vi "Queue Driver-Receive.vi"(0 "States[]":string[](array[string]), 5 "Data":variant, 7 "Queue Name":string, 11 "Error In":errorcluster, 13 "Queue Operation":T2) -> (4 "Dequeue Element":T1, 15 "Error Out":errorcluster)   [LabVIEW 2020]
doc: "The VI performs the queue operations. The operations include create, enqueue, dequeue, flush and closes the queue."
uses:
  Controls/Queue Element.ctl
  Controls/Queue Operation.ctl
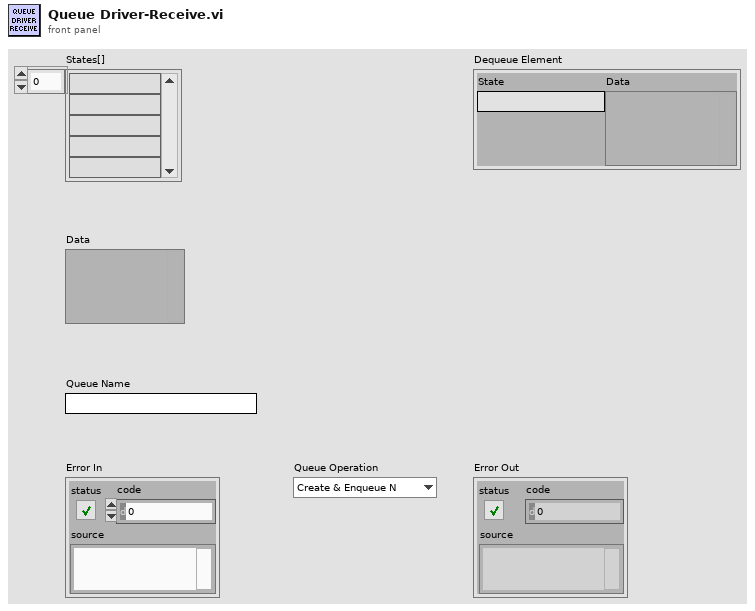
[diagram p1: front panel]
types:
  T1 = typedef "Queue Element.ctl" = cluster{"State":string, "Data":variant}
  T2 = typedef "Queue Operation.ctl" = enum16{"Create & Enqueue N", "Enqueue N", "Dequeue", "Enstack N", "Flush", "Release"}
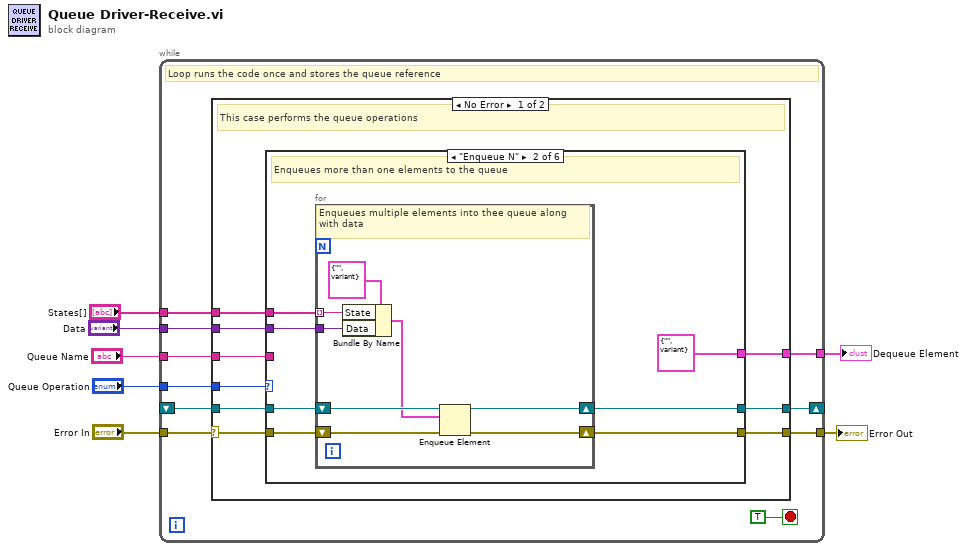
[diagram p0: block diagram]
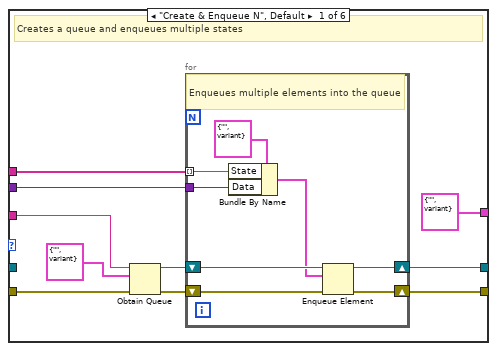
[diagram p2: hidden frame]
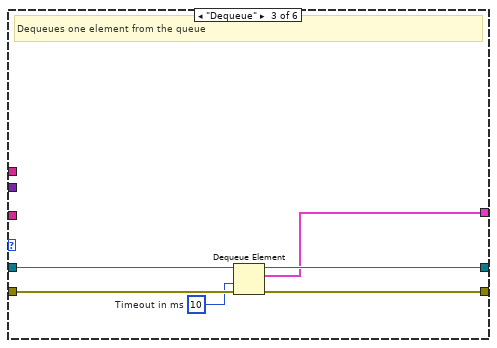
[diagram p3: hidden frame]
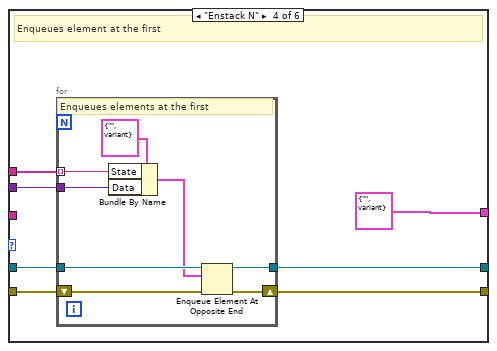
[diagram p4: hidden frame]
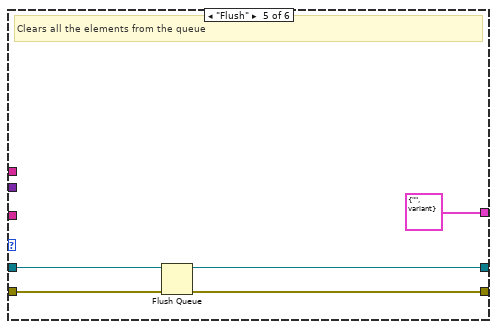
[diagram p5: hidden frame]
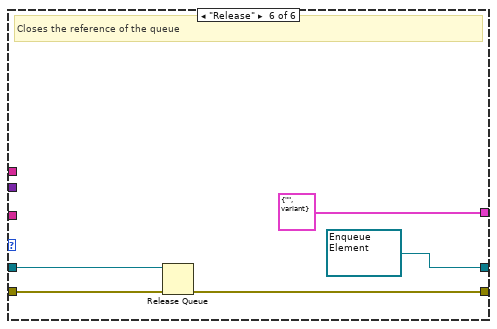
[diagram p6: hidden frame]
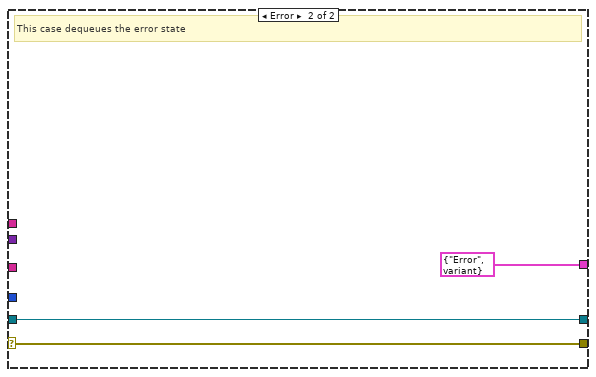
[diagram p7: hidden frame]
diagram:
  n1 = while {
    tunnel: "Error In" -> [w17]
    tunnel: "Queue Operation" -> [w16]
    tunnel: "Queue Name" -> [w15]
    shift-right: [w14] -> _
    shift-left: _ -> [w13]
    tunnel: [w12] -> w4
    tunnel: [w10] -> w3
    tunnel: "Data" -> [w9]
    tunnel: "States[]" -> [w8]
    stop <- TRUE stop-if-true
    # "Loop runs the code once and stores the queue reference"
    n2 = case shown="No Error" w17 {
      selector: w17 -> [w26 w92]
      tunnel: w16 -> [w25 _]
      tunnel: w15 -> [w24 _]
      tunnel: [w23 w93] -> w14
      tunnel: w13 -> [w22 w93]
      tunnel: [w21 w92] -> w12
      tunnel: [w20 T1 {"State"="Error", "Data"=variant} ("Dequeue Element")] -> w10
      tunnel: w9 -> [w19 _]
      tunnel: w8 -> [w18 _]
      frame No Error {
        # "This case performs the queue operations"
        n3 = case shown="\"Enqueue N\"" w25 {
          tunnel: [w30 w50 w64 w71 w84 w89] -> w21
          tunnel: w26 -> [w36 w51 w65 w72 w85 w90]
          tunnel: w24 -> [w35 _ _ _ _ _]
          tunnel: [w31 w49 w63 w69 w82 refnum<queue> refnum ("queue out")] -> w23
          tunnel: w22 -> [_ w46 w62 w70 w83 w88]
          tunnel: [T1 {"State"="", "Data"=variant} ("Dequeue Element") T1 {"State"="", "Data"=variant} ("Dequeue Element") w60 T1 {"State"="", "Data"=variant} ("Dequeue Element") T1 {"State"="", "Data"=variant} ("Dequeue Element") T1 {"State"="", "Data"=variant} ("Dequeue Element")] -> w20
          tunnel: w19 -> [w27 w45 _ w66 _ _]
          tunnel: w18 -> [w28 w47 _ w68 _ _]
          frame "Create & Enqueue N", Default {
            # "Creates a queue and enqueues multiple states"
            n4 = Obtain Queue(name (unnamed)=w35, element data type=T1 {"State"="", "Data"=variant} ("Dequeue Element"), error in (no error)=w36) -> (queue out=w32:refnum<queue>, error out=w29:errorcluster)  [unwired: 2 in, 1 out]
            n5 = for {
              shift-right: [w43] -> w30
              shift-left: w29 -> [w44]
              tunnel: w28 -> [w38] mode=indexing
              shift-right: [w41] -> w31
              shift-left: w32 -> [w42]
              tunnel: w27 -> [w37]
              # "Enqueues multiple elements into the queue"
              n6 = Bundle By Name(cluster=T1 {"State"="", "Data"=variant} ("Dequeue Element"), "State"=w38, "Data"=w37) -> (w40:T1)
              n7 = Enqueue Element(queue=w42, element=w40, error in (no error)=w44) -> (queue out=w41:refnum<queue>, error out=w43:errorcluster)  [unwired: 1 in, 1 out]
            }
          }
          frame "Enqueue N" {
            # "Enqueues more than one elements to the queue"
            n8 = for {
              shift-right: [w58] -> w50
              shift-left: w51 -> [w59]
              tunnel: w47 -> [w53] mode=indexing
              shift-right: [w56] -> w49
              shift-left: w46 -> [w57]
              tunnel: w45 -> [w52]
              # "Enqueues multiple elements into thee queue along with data"
              n9 = Bundle By Name(cluster=T1 {"State"="", "Data"=variant} ("Dequeue Element"), "State"=w53, "Data"=w52) -> (w55:T1)
              n10 = Enqueue Element(queue=w57, element=w55, error in (no error)=w59) -> (queue out=w56:refnum<queue>, error out=w58:errorcluster)  [unwired: 1 in, 1 out]
            }
          }
          frame "Dequeue" {
            w61 = 10  # Timeout in ms
            # "Dequeues one element from the queue"
            n11 = Dequeue Element(queue=w62, timeout in ms (-1)=w61, error in (no error)=w65) -> (queue out=w63:refnum<queue>, element=w60:T1, error out=w64:errorcluster)  [unwired: 1 out]
          }
          frame "Enstack N" {
            # "Enqueues element at the first"
            n12 = for {
              tunnel: w70 -> [w78]
              tunnel: [w77] -> w69
              shift-right: [w79] -> w71
              shift-left: w72 -> [w80]
              tunnel: w68 -> [w74] mode=indexing
              tunnel: w66 -> [w73]
              # "Enqueues elements at the first"
              n13 = Bundle By Name(cluster=T1 {"State"="", "Data"=variant} ("Enqueue Element"), "State"=w74, "Data"=w73) -> (w76:T1)
              n14 = Enqueue Element At Opposite End(queue=w78, element=w76, error in (no error)=w80) -> (queue out=w77:refnum<queue>, error out=w79:errorcluster)  [unwired: 1 in, 1 out]
            }
          }
          frame "Flush" {
            # "Clears all the elements from the queue"
            n15 = Flush Queue(queue=w83, error in (no error)=w85) -> (queue out=w82:refnum<queue>, error out=w84:errorcluster)  [unwired: 1 out]
          }
          frame "Release" {
            # "Closes the reference of the queue"
            n16 = Release Queue(queue=w88, error in (no error)=w90) -> (error out=w89:errorcluster)  [unwired: 1 in, 2 out]
          }
        }
      }
      frame Error {
        # "This case dequeues the error state"
      }
    }
  }
  "Error Out" <- w4
  "Dequeue Element" <- w3
